vi "3. Get Time References.vi"() -> ()   [LabVIEW 2019]
doc: "Demonstrates how to monitor all time references running on a real-time system."
uses:
  <instrlib>/niSync/niSync.llb/niSync Initialize (Default).vi
panel:
  in  "NI-Sync Resource":tag
  out "Error Out":errorcluster
  out "Table":string[][](table)
  # "Overview: Demonstrates how to monitor all time references running on a real-time system.\nRequirements: Runs on Windows and LinuxRT hosts to monitor LinuxRT devices.\nInstructions:\n1. Select the real-time system to monitor/configure in the NI-Sync Resource control.\n2. Run the VI to get information on the time references running on that system."
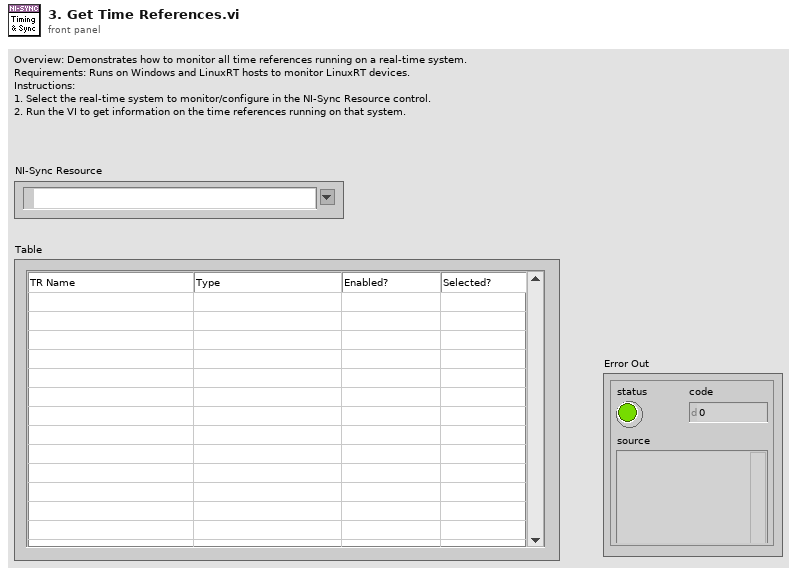
[diagram p1: front panel]
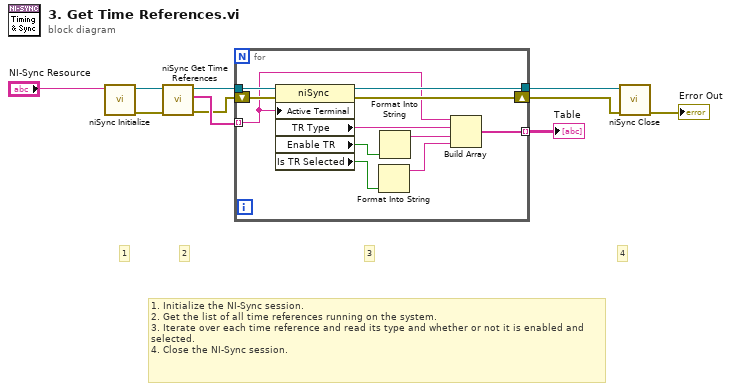
[diagram p0: block diagram]
diagram:
  # "1. Initialize the NI-Sync session.\n2. Get the list of all time references running on the system.\n3. Iterate over each time reference and read its type and whether or not it is enabled and selected.\n4. Close the NI-Sync session."
  # "4"
  # "3"
  # "2"
  # "1"
  n1 = call-poly <instrlib>:"niSync Initialize.vi"("resource name"="NI-Sync Resource") -> ("error out"=w9:errorcluster, "instrument handle out"=w10:refnum<k15>)  [unwired: 9 in]
  n2 = call <instrlib>:"niSync Get Time References.vi"("error in (no error)"=w9, "instrument handle"=w10) -> ("error out"=w6:errorcluster, "time references"=w7:string[], "instrument handle out"=w8:refnum<k15>)  [unwired: 7 in]
  n3 = for {
    tunnel: w8 -> [w21]
    tunnel: w7 -> [w17] mode=indexing
    tunnel: [w19] -> w4
    shift-right: [w18] -> w3
    shift-left: w6 -> [w20]
    tunnel: [w13] -> w5 mode=indexing
    n4 = property class="niSync"(reference=w21, error in=w20, "Active Terminal"=w17) -> (reference out=w19:refnum<k15>, error out=w18:errorcluster, "TR Type"=w16:string, "Enable TR"=w11:bool, "Is TR Selected"=w15:bool)
    n5 = Format Into String(w15) -> (resulting string=w14:string)  [unwired: 3 in, 1 out]
    n6 = Format Into String(w11) -> (resulting string=w12:string)  [unwired: 3 in, 1 out]
    n7 = Build Array(w17, w16, w12, w14) -> (w13:string[])
  }
  "Table" <- w5
  n8 = call <instrlib>:"niSync Close.vi"("error in (no error)"=w3, "instrument handle"=w4) -> ("error out"=→"Error Out":errorcluster)  [unwired: 9 in]
